vi "小三轮的 I2C Get Configuration.vi"(9 "Configuration":u8, 10 "Control":u8, 11 "Address In":u8) -> (2 "ACK":bool, 3 "I2C Configuration":T1)   [LabVIEW 2017]
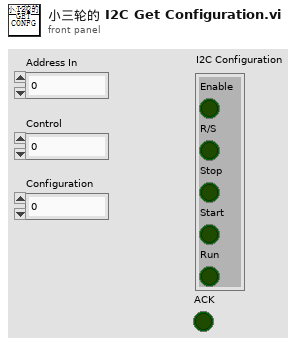
[diagram p1: front panel]
types:
  T1 = typedef "小三轮的 I2C Configuration.ctl" = cluster{"Enable":bool, "R/S":bool, "Stop":bool, "Start":bool, "Run":bool}
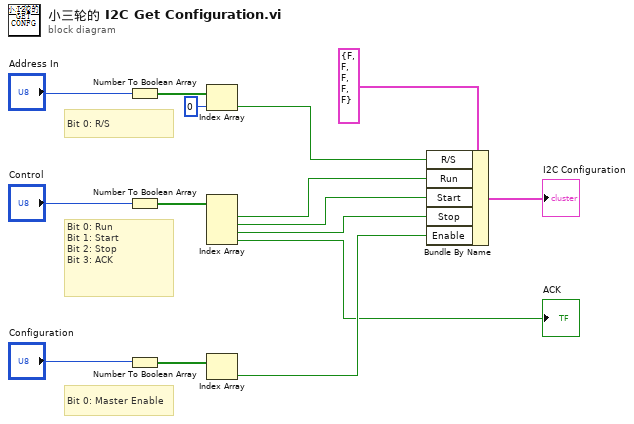
[diagram p0: block diagram]
diagram:
  # "Bit 0: R/S"
  # "Bit 0: Run \nBit 1: Start\nBit 2: Stop\nBit 3: ACK"
  # "Bit 0: Master Enable"
  n1 = Number To Boolean Array(number="Address In") -> (Boolean array=w12:bool[])
  n2 = Number To Boolean Array(number="Control") -> (Boolean array=w8:bool[])
  n3 = Number To Boolean Array(number="Configuration") -> (Boolean array=w6:bool[])
  n4 = Index Array(array=w12, index=0) -> (element=w10:bool)
  n5 = Index Array(array=w8) -> (element #1=w5:bool, element #2=w4:bool, element #3=w3:bool, element #4=→"ACK":bool)  [unwired: 4 in]
  n6 = Index Array(array=w6) -> (element=w2:bool)  [unwired: 1 in]
  n7 = Bundle By Name(cluster=T1 {"Enable"=FALSE, "R/S"=FALSE, "Stop"=FALSE, "Start"=FALSE, "Run"=FALSE} ("I2C Configuration"), "R/S"=w10, "Run"=w5, "Start"=w4, "Stop"=w3, "Enable"=w2) -> (→"I2C Configuration":T1)
